vi "二维数组排序.vi"() -> ()   [LabVIEW 2020]
panel:
  out "转回二维数组":i32[][](array[numeric])
  out "排序后的一维数组":u32[](array[numeric])
  out "转换为一维数组":u32[](array[numeric])
  out "原始二维数组":u32[][](array[numeric])
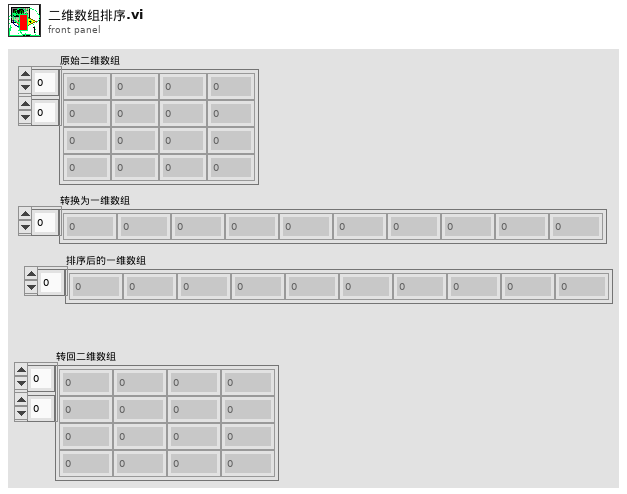
[diagram p1: front panel]
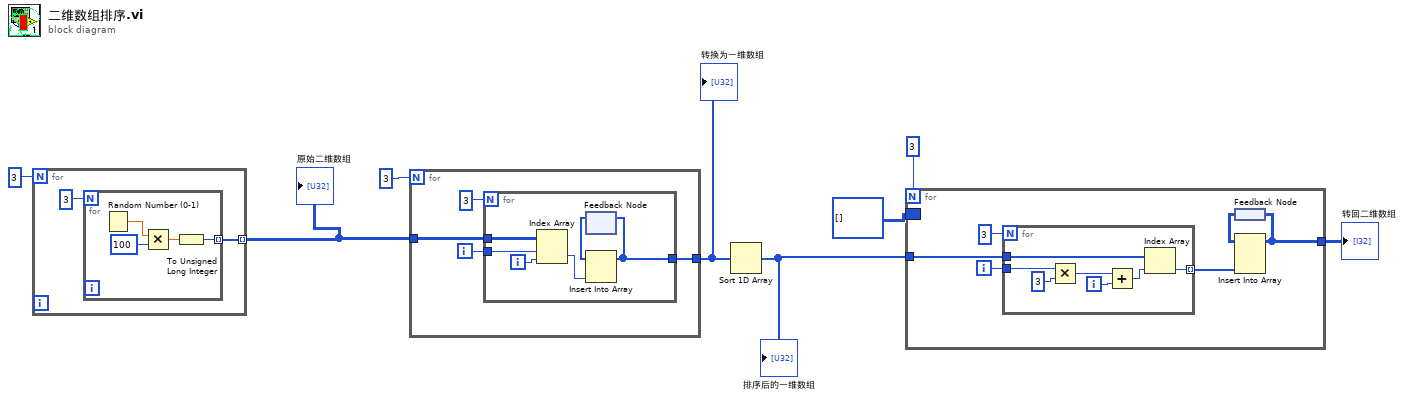
[diagram p0: block diagram]
diagram:
  n1 = for {
    N: 3 -> [_]
    tunnel: [w9] -> w1 mode=indexing
    n2 = for {
      N: 3 -> [_]
      tunnel: [w11] -> w9 mode=indexing
      n3 = Random Number (0-1)() -> (number: 0 to 1=w14:dbl)
      n4 = Multiply(x=w14, y=100) -> (x*y=w12:dbl)
      n5 = To Unsigned Long Integer(number=w12) -> (unsigned 32bit integer=w11:u32)
    }
  }
  "原始二维数组" <- w1
  n6 = for {
    N: 3 -> [_]
    tunnel: w1 -> [w17]
    tunnel: [w15] -> w6
    i -> [w16]
    n7 = for {
      N: 3 -> [_]
      tunnel: w17 -> [w24]
      tunnel: w16 -> [w23]
      tunnel: [w19] -> w15
      i -> [w22]
      n8 = Index Array(array=w24, index (row)=w23, index (col)=w22) -> (element=w21:u32)
      n9 = feedback #1() -> (w20:u32[])  [unwired: 1 in]
      n10 = Insert Into Array(array=w20, new element=w21) -> (w19:u32[])  [unwired: 1 in]
      n11 = feedback-in #1(w19) -> ()
    }
  }
  "转换为一维数组" <- w6
  n12 = Sort 1D Array(array=w6) -> (sorted array=w4:u32[])
  "排序后的一维数组" <- w4
  n13 = for {
    N: 3 -> [_]
    tunnel: w4 -> [w29]
    tunnel: [w25] -> w3
    border: i32[][] [] -> [_]
    i -> [w28]
    n14 = for {
      N: 3 -> [_]
      tunnel: w29 -> [w37]
      tunnel: w28 -> [w35]
      tunnel: [w36] -> w27 mode=indexing
      i -> [w33]
      n15 = Multiply(x=w35, y=3) -> (x*y=w32:i32)
      n16 = Add(x=w32, y=w33) -> (x+y=w31:i32)
      n17 = Index Array(array=w37, index=w31) -> (element=w36:u32)
    }
    n18 = feedback #2() -> (w26:i32[][])
    n19 = Insert Into Array(array=w26, new element=w27) -> (w25:i32[][])  [unwired: 2 in]
    n20 = feedback-in #2(w25) -> ()
  }
  "转回二维数组" <- w3
